vi "Control - Diesel - Fuel Command Host.vi"() -> ()   [LabVIEW 2015, in "ECS-Host.lvlib"]
uses:
  ECS-Host.lvlib
  <vilib>/addons/Software Calibration Management/XControls/TBL2D.xctl
  <vilib>/addons/Software Calibration Management/XControls/SubHost.xctl
panel:
  in  "Fuel Cut":T1(xcontrol)
  in  "Smoke Limit":T1(xcontrol)
  in  "Fuel_ManE":bool
  in  "Fuel_Man":sgl caption="[mg/cyc]"
  out "Fuel_Des":sgl caption="[mg/cyc]"
  out "Fuel_FFTblOut":sgl caption="[mg/cyc]"
  in  "Fuel_FFTbl":cluster{"X":sgl[], "Y":sgl[], "Z":sgl[][]}(xcontrol)
  # "Fuel Calibration"
  # "SubHosts"
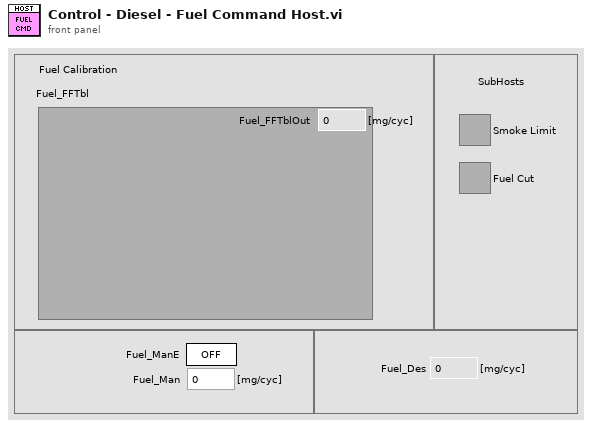
[diagram p1: front panel]
types:
  T1 = cluster{"Name":string, "Host VI":path, "Pairing File":path, "Display Name":string}
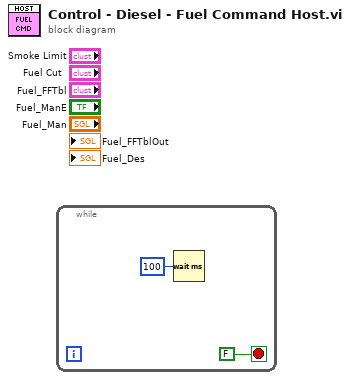
[diagram p0: block diagram]
diagram:
  n1 = while {
    stop <- FALSE stop-if-true
    n2 = Wait (ms)(milliseconds to wait=u32 100) -> ()  [unwired: 1 out]
  }
